vi "Main_FPGA.vi"() -> ()   [LabVIEW 2018]
uses:
  <vilib>/rvi/eio/common/nirviEmuTemplateMethod_errors.vi
  <vilib>/rvi/Emulation/niFpgaGetClockAttributes.vi
  <vilib>/rvi/Emulation/niFpgaSctlEmulationGetInTimedLoop.vi
  <vilib>/rvi/Emulation/niFpgaEmulationReportErrorSimple.vi
  <vilib>/rvi/Emulation/niFpgaProcessEmulError.vi
  <vilib>/rvi/Emulation/niFpgaCriticalErrorInLSC.vi
  <vilib>/eio/EIONode/EIONode.xnode
  <vilib>/addons/control/pid/fpga.llb/XNode/niFpgaPID.xnode
panel:
  in  "Mod7/13 Intercooler in temp":fxp<+/-,20,5>
  out "Mod6/Unit L":bool
  out "Mod6/Unit R":bool
  out "Mod8/AI15":fxp<+/-,24,5>
  out "Mod8/AI5":fxp<+/-,24,5>
  out "Mod8/AI4":fxp<+/-,24,5>
  out "Speed_cmd":fxp<+/-,17,6>
  in  "FeedFw_Ena":bool
  in  "ACC_FeedFw":fxp<+/-,16,5>
  out "Acc_2":fxp<+/-,36,10>
  out "Acc_1":fxp<+/-,36,10>
  in  "E-Acc_2":T1={"Gain"=1.0, "OffSet"=0.0}
  in  "E-Acc_1":T1={"Gain"=1.0, "OffSet"=0.0}
  in  "Speed Control Soll (%)":fxp<+/-,16,5>
  in  "Parameter Speed Control":fxp<+/-,16,5>
  in  "PID gains":T2={"proportional gain (Kc)"=1.5, "integral gain (Kc*Ts/Ti)"=0.19921875, "derivative gain (Kc*Td/Ts)"=0.0}
  in  "output range":T3={"output high"=10.0, "output low"=0.0}
  in  "Regler Speed Control":bool
  in  "Ist Speed Control":fxp<+/-,16,5>
  in  "Count (mSec) Fahrhebel":u32=25
  out "Tick Count(mSec) Hydraulic Wave":u32
  out "Count Hydraulic  Wave":i64
  out "Mod6/Fuel Transmitter":bool
  out "Mod6/DI30":bool
  out "Tick Count(mSec) Hydraulic":u32
  out "Count Hydraulic":i64
  in  "Mod7/Hydraulic clutch Set point":fxp<+/-,20,5>
  in  "Mod7/Hydraulic pump actuator Soll":fxp<+/-,20,5>
  in  "Mod7/Out 2":fxp<+/-,20,5>
  in  "Mod7/Out 1":fxp<+/-,20,5>
  out "DM Count":i64
  out "Tick Count(mSec)":u32
  in  "Mod4/DO30":bool
  in  "Mod4/Release Brake M":bool
  in  "Mod4/Richtung Engine Speed M":bool
  in  "Mod4/Release Engine Speed M":bool
  in  "Mod4/Richtung Up M":bool
  in  "Mod4/Release Up M":bool
  out "Mod6/End Position DOWN M":bool
  out "Mod6/DOWN M":bool
  out "Mod6/UP M":bool
  out "Mod6/End Position UP M":bool
  in  "Mod7/Up M Set point":fxp<+/-,20,5>
  in  "Mod7/Torque M Set point":fxp<+/-,20,5>
  out "Mod8/Engine Speed M":fxp<+/-,24,5>
  out "Mod8/Up M":fxp<+/-,24,5>
  in  "Mod4/Clutch":bool
  in  "Mod4/Temperature Control Release":bool
  in  "Mod4/Temperature Control OFF":bool
  in  "Mod4/Calibration ON Brake H":bool
  in  "Mod4/Unit ON Brake H":bool
  in  "Mod4/Brake Performance ON Brake H":bool
  in  "Mod4/Control Reset Brake H":bool
  in  "Mod4/Control ON Brake H":bool
  in  "Mod4/Oil ON":bool
  in  "Mod3/Calibration Brake R":bool
  in  "Mod3/Unit ON Brake R":bool
  in  "Mod3/Brake Performance ON Brake R":bool
  in  "Mod3/Control Reset Brake R":bool
  in  "Mod3/Control ON Brake R":bool
  in  "Mod3/Horn":bool
  in  "Mod3/DO20":bool
  in  "Mod3/Speed Control Release":bool
  in  "Mod3/DO18":bool
  in  "Mod3/Flashing light":bool
  in  "Mod3/Calibration ON Brake L":bool
  in  "Mod3/Unit ON Brake L":bool
  in  "Mod3/Brake Performance ON Brake L":bool
  in  "Mod3/Control Reset Brake L":bool
  in  "Mod3/Control ON Brake L":bool
  in  "Mod3/Converter Clutch ON":bool
  in  "Mod3/Fuel Pump ON":bool
  in  "Mod3/Engine Ignition ON":bool
  in  "Mod3/Start Engine":bool
  in  "Mod3/Engine Pre Glow ON":bool
  in  "Cooling  Set point (°C)":fxp<+/-,16,5>
  in  "Heater Set point (°C)":fxp<+/-,16,5>
  in  "Alarm 24 ON":bool
  in  "Alarm 23 ON":bool
  in  "Alarm 22 ON":bool
  in  "Alarm 21 ON":bool
  in  "Alarm 20 ON":bool
  in  "Alarm 19 ON":bool
  in  "Alarm 18 ON":bool
  in  "Alarm 17 ON":bool
  in  "Alarm 16 ON":bool
  in  "Alarm 15 ON":bool
  in  "Alarm 14 ON":bool
  in  "Alarm 13 ON":bool
  in  "Alarm 12 ON":bool
  in  "Alarm 11 ON":bool
  in  "Alarm 10 ON":bool
  in  "Alarm 9 ON":bool
  in  "Alarm 8 ON":bool
  in  "Alarm 7 ON":bool
  in  "Alarm 6 ON":bool
  in  "Alarm 5 ON":bool
  in  "Alarm 4 ON":bool
  in  "Alarm 3 ON":bool
  out "Alarm":bool
  in  "Alarm 2 ON":bool
  in  "Alarm 1 ON":bool
  in  "Alarm ON":bool
  in  "STOP":bool
  out "Mod8/Kal 2 Brake H":fxp<+/-,24,5>
  out "Mod8/Kal 1 Brake H":fxp<+/-,24,5>
  out "Mod8/Kal 2 Brake R":fxp<+/-,24,5>
  out "Mod8/Kal 1 Brake R":fxp<+/-,24,5>
  out "Mod8/Kal 2 Brake L":fxp<+/-,24,5>
  out "Mod8/Kal 1 Brake L":fxp<+/-,24,5>
  out "Mod8/Engine Speed Wave Sensor":fxp<+/-,24,5>
  out "Mod8/Speed Control":fxp<+/-,24,5>
  out "Mod8/Torque  H":fxp<+/-,24,5>
  out "Mod8/Torque  R":fxp<+/-,24,5>
  out "Mod8/Torque  L":fxp<+/-,24,5>
  in  "Mod3/System Reset/ON":bool
  out "Mod6/Clutch open":bool
  out "Mod6/Clutch closed":bool
  out "Mod6/Alarm 25 Basement":bool
  out "Mod6/Unit L-R":bool
  out "Mod6/Unit H":bool
  out "Mod6/Unit H-L-R":bool
  out "Mod6/Sytem Ready":bool
  out "Mod6/Watchdog Ready":bool
  out "Mod6/Alarm 2 Brake back":bool
  out "Mod6/Alarm 1 Brake back":bool
  out "Mod6/Temperature Brake back":bool
  out "Mod6/Ready Brake back":bool
  out "Mod6/Error Brake back":bool
  out "Mod6/Alarm 24 Overload Warning Oil Heating":bool
  out "Mod6/Alarm 23 Overload Warning Oil Pump":bool
  out "Mod6/Alarm 22 max Oil Pressure":bool
  out "Mod6/Alarm 21 min Oil Pressure":bool
  out "Mod6/Alarm 20 max Oil Temperature":bool
  out "Mod6/Alarm 18 Oil Level":bool
  out "Mod6/Alarm 19 min Oil Pressure":bool
  out "Mod6/Alarm 17 Oil Pressure Difference":bool
  out "Mod5/Alarm 2 Brake R":bool
  out "Mod5/Alarm 1 Brake R":bool
  out "Mod5/Temperature Brake R":bool
  out "Mod5/Ready Brake R":bool
  out "Mod5/Error Brake R":bool
  out "Mod5/Alarm 16 Fundament 4":bool
  out "Mod5/Alarm 15 Fundament 3":bool
  out "Mod5/Alarm 14 Fundament 2":bool
  out "Mod5/Alarm 13 Fundament 1":bool
  out "Mod5/Alarm 12 Spring Element":bool
  out "Mod5/Alarm 11 Watchdog":bool
  out "Mod5/Alarm 10 Fuel Depot":bool
  out "Mod5/Alarm 9 IGBT_ON":bool
  out "Mod5/Alarm 2 Brake L":bool
  out "Mod5/Alarm 1 Brake L":bool
  out "Mod5/Temperature Brake L":bool
  out "Mod5/Ready Brake L":bool
  out "Mod5/Error Brake L":bool
  out "Mod5/Alarm 8 Cooling Water":bool
  out "Mod5/Alarm 7 Exhaust":bool
  out "Mod5/Alarm 6 CO2":bool
  out "Mod5/Alarm 5 Clutch":bool
  out "Mod5/Alarm 4 Speed Control":bool
  out "Mod5/Alarm 3 Flow Control Unit":bool
  out "Mod5/Alarm 2 Gas":bool
  out "Mod5/Alarm 1 Fire":bool
  out "Mod2/Engine Speed  H":fxp<+/-,20,5>
  out "Mod2/Engine Speed R":fxp<+/-,20,5>
  out "Mod2/Engine Speed  L":fxp<+/-,20,5>
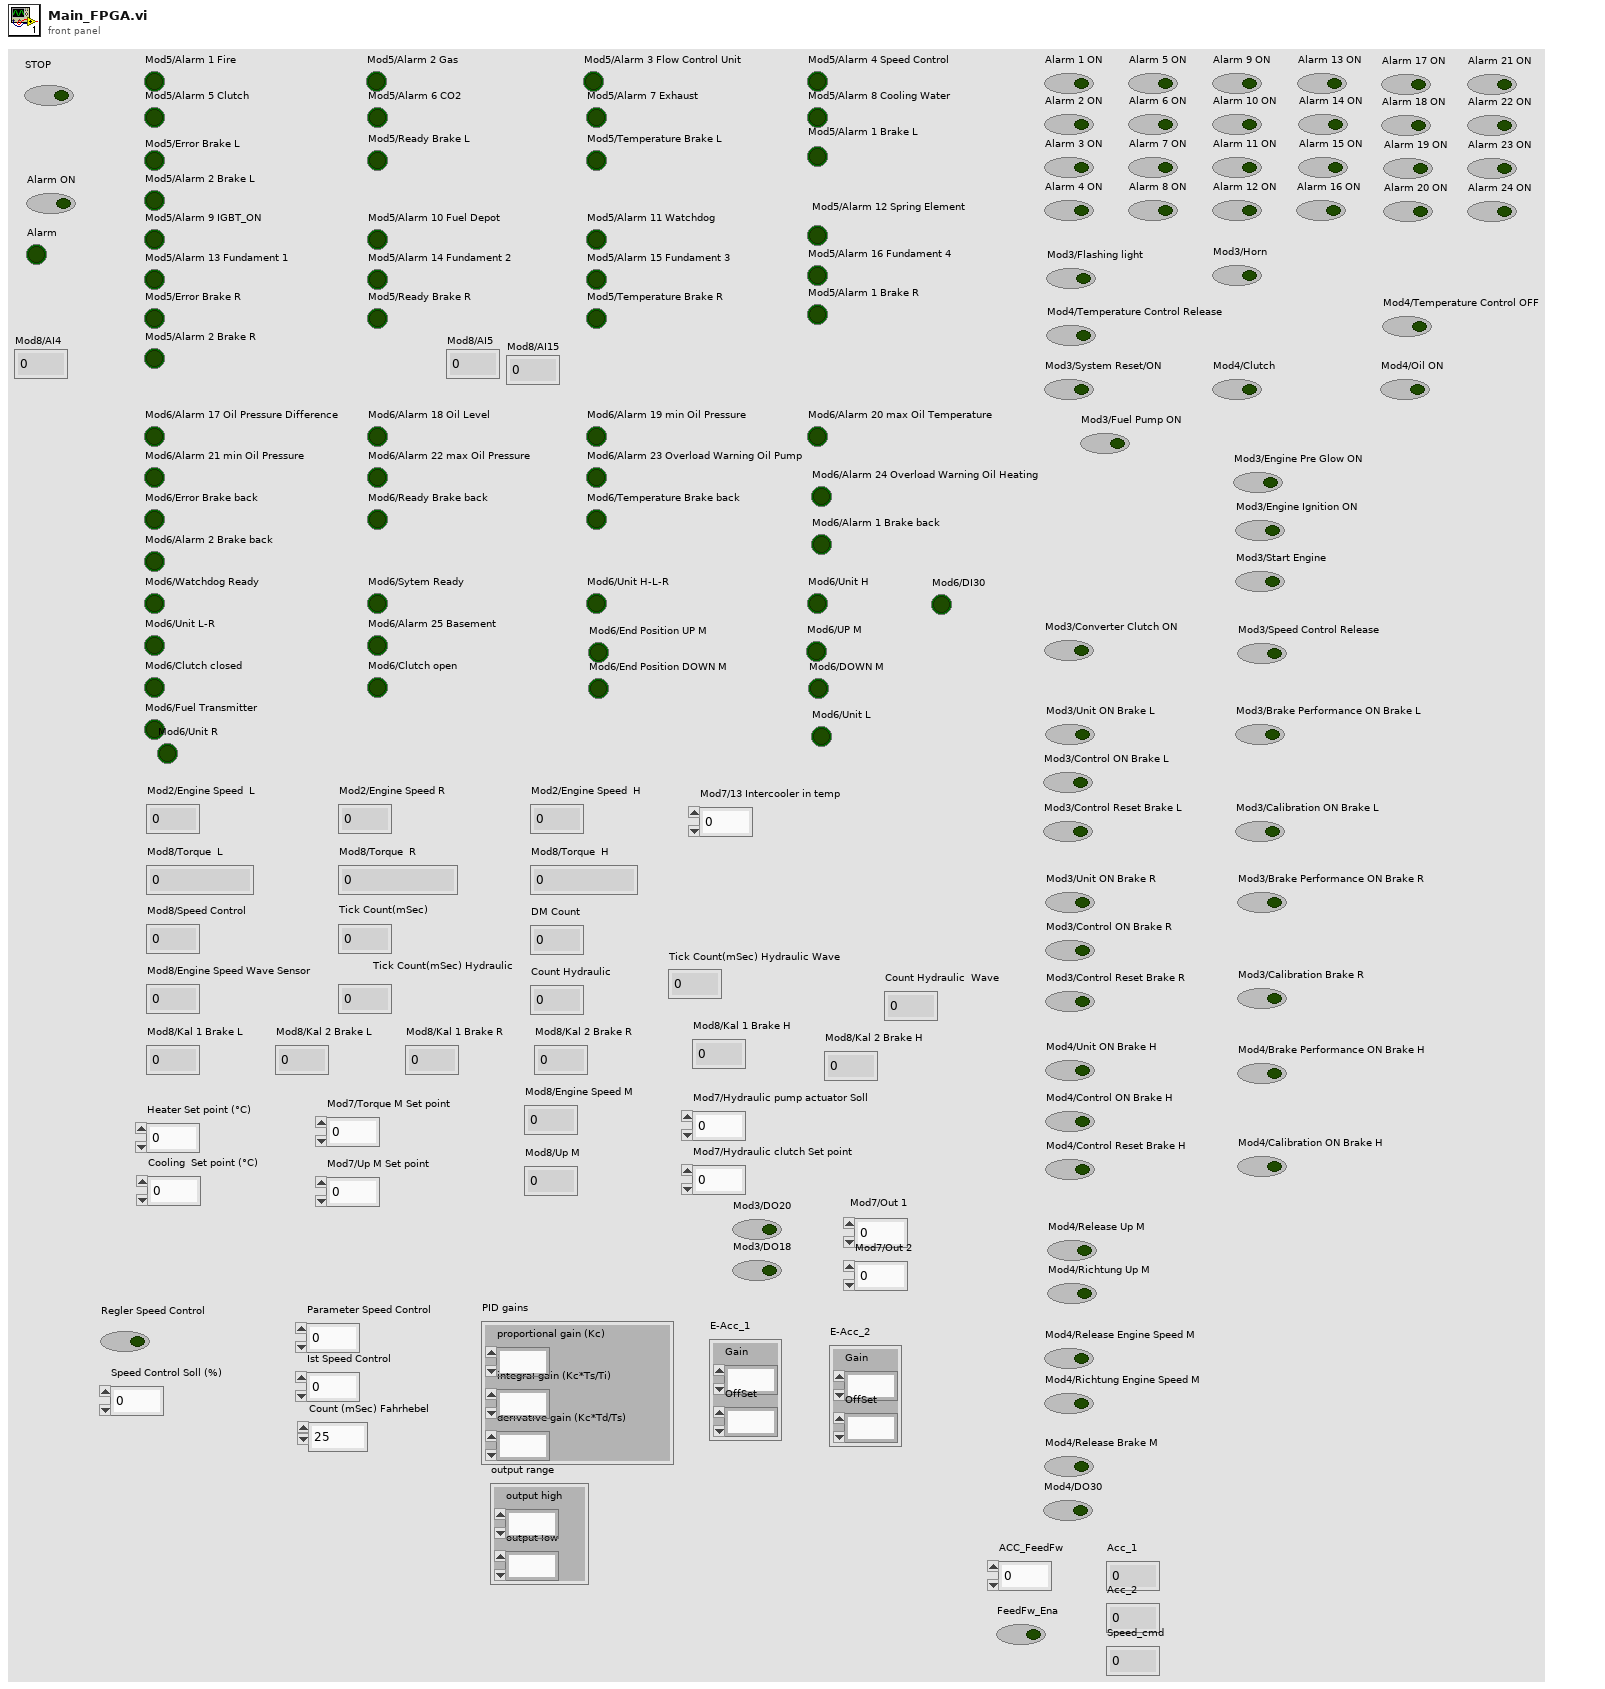
[diagram p1: front panel]
types:
  T1 = cluster{"Gain":fxp<+/-,20,5>, "OffSet":fxp<+/-,20,5>}
  T2 = cluster{"proportional gain (Kc)":fxp<+/-,16,8>, "integral gain (Kc*Ts/Ti)":fxp<+/-,16,8>, "derivative gain (Kc*Td/Ts)":fxp<+/-,16,8>}
  T3 = cluster{"output high":fxp<+/-,16,5>, "output low":fxp<+/-,16,5>}
  T4 = cluster{"proportional gain (Kc)":i16, "integral gain (Kc*Ts/Ti)":i16, "derivative gain (Kc*Td/Ts)":i16}
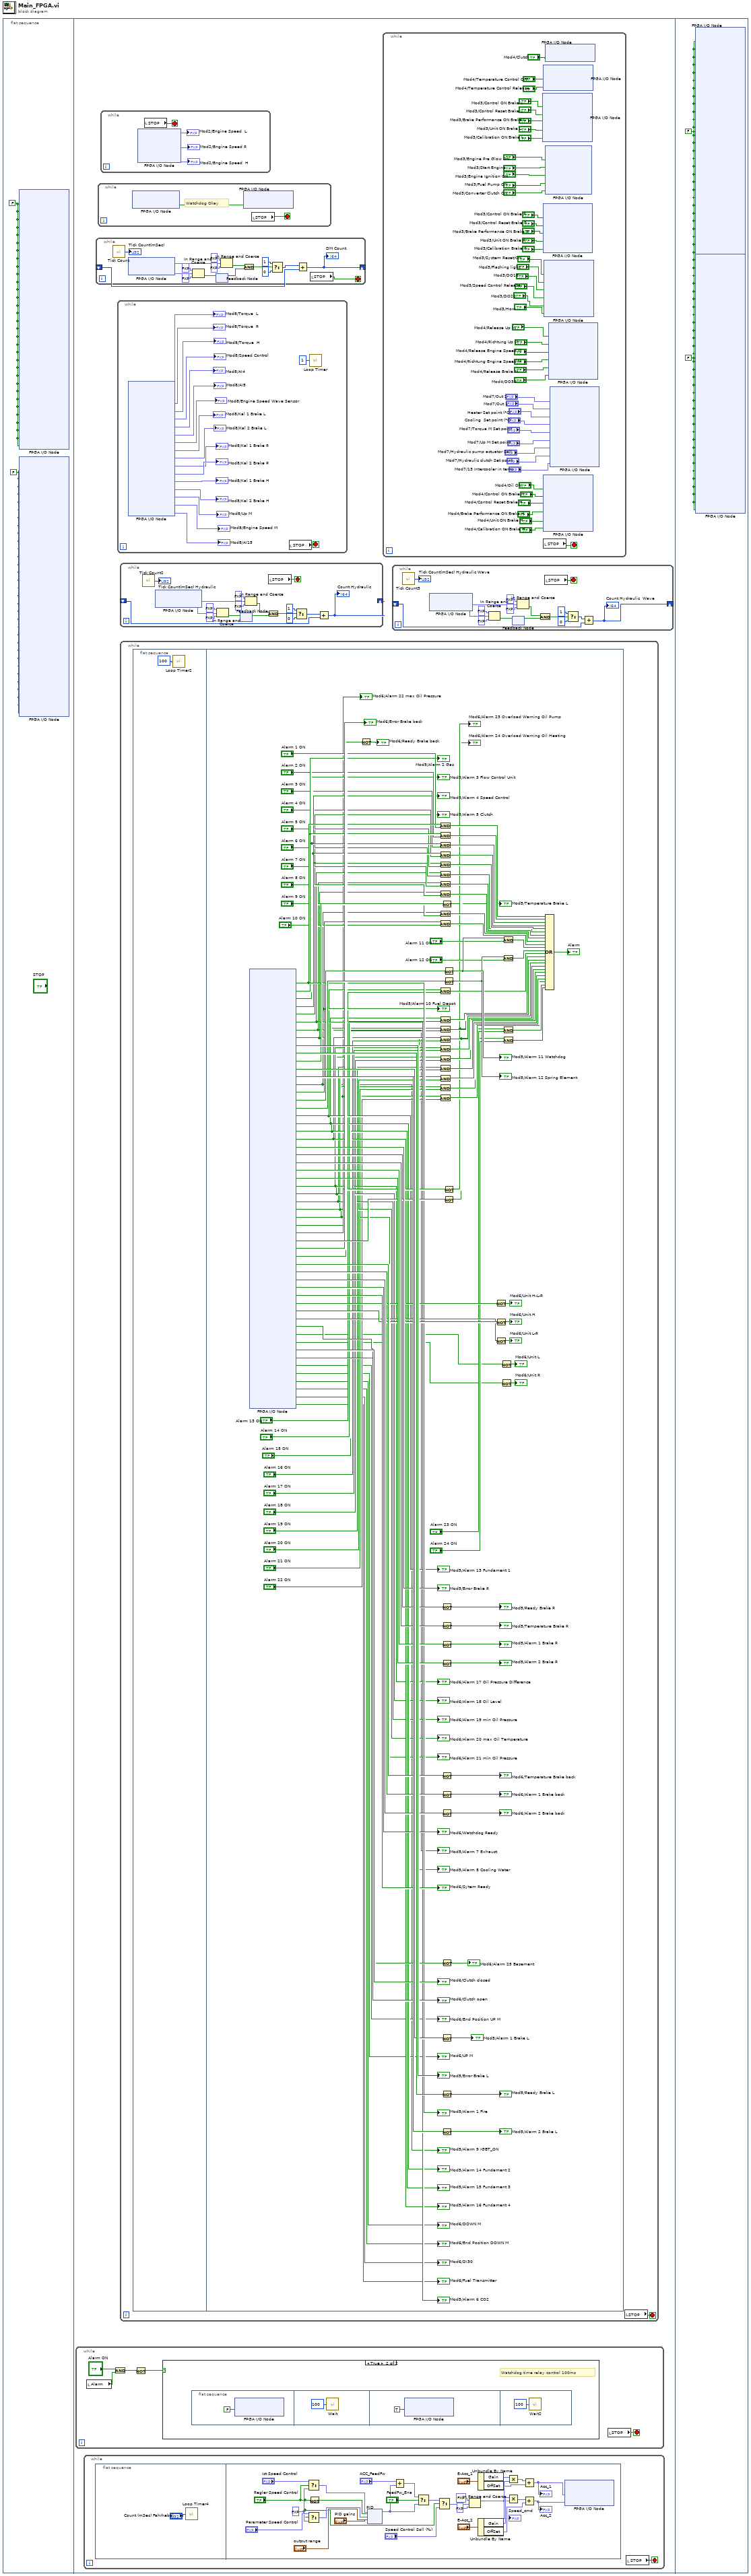
[diagram p0: block diagram]
diagram:
  n1 = flat-sequence {
    frame #0 {
      w1 = FALSE ("Mod4/DO0")
      w2 = FALSE ("Mod3/DO0")
      n2 = xnode "FPGA I/O Node"("Mod4/DO0"=w1, "Mod4/DO1"=w1, "Mod4/DO2"=w1, "Mod4/DO3"=w1, "Mod4/DO4"=w1, "Mod4/DO5"=w1, "Mod4/DO6"=w1, "Mod4/DO7"=w1, "Mod4/DO8"=w1, "Mod4/DO9"=w1, "Mod4/DO10"=w1, "Mod4/DO11"=w1, "Mod4/DO12"=w1, "Mod4/DO13"=w1, "Mod4/DO14"=w1, "Mod4/DO15"=w1, "Mod4/DO16"=w1, "Mod4/DO17"=w1, "Mod4/DO18"=w1, "Mod4/DO19"=w1, "Mod4/DO20"=w1, "Mod4/DO21"=w1, "Mod4/DO22"=w1, "Mod4/DO23"=w1, "Mod4/DO24"=w1, "Mod4/DO25"=w1, "Mod4/DO26"=w1, "Mod4/DO27"=w1, "Mod4/DO28"=w1, "Mod4/DO29"=w1, "Mod4/DO30"=w1, "Mod4/DO31"=w1) -> ()  [unwired: 32 in, 32 out]
      n3 = xnode "FPGA I/O Node"("Mod3/DO0"=w2, "Mod3/DO1"=w2, "Mod3/DO2"=w2, "Mod3/DO3"=w2, "Mod3/DO4"=w2, "Mod3/DO5"=w2, "Mod3/DO6"=w2, "Mod3/DO7"=w2, "Mod3/DO8"=w2, "Mod3/DO9"=w2, "Mod3/DO10"=w2, "Mod3/DO11"=w2, "Mod3/DO12"=w2, "Mod3/DO13"=w2, "Mod3/DO14"=w2, "Mod3/DO15"=w2, "Mod3/DO16"=w2, "Mod3/DO17"=w2, "Mod3/DO18"=w2, "Mod3/DO19"=w2, "Mod3/DO20"=w2, "Mod3/DO21"=w2, "Mod3/DO22"=w2, "Mod3/DO23"=w2, "Mod3/DO24"=w2, "Mod3/DO25"=w2, "Mod3/DO26"=w2, "Mod3/DO27"=w2, "Mod3/DO28"=w2, "Mod3/DO29"=w2, "Mod3/DO30"=w2, "Mod3/DO31"=w2) -> ()  [unwired: 32 in, 32 out]
    }
    frame #1 {
      n4 = while {
        stop <- w178 stop-if-true
        n5 = local read "Alarm"() -> (w181:bool)
        n6 = And(x="Alarm ON", y=w181) -> (x .and. y?=w180:bool)
        n7 = Not(x=w180) -> (.not. x?=w179:bool)
        n8 = case shown="True" w179 {
          frame False {
          }
          frame True {
            # "Watchdog time relay control 100ms"
            n9 = flat-sequence {
              frame #0 {
                n10 = xnode "FPGA I/O Node"("Mod4/DO16"=FALSE) -> ()  [unwired: 1 in, 1 out]
              }
              frame #1 {
                n11 = call "Wait"("Count(mSec)"=u32 100) -> ()  [unwired: 1 out]
              }
              frame #2 {
                n12 = xnode "FPGA I/O Node"("Mod4/DO16"=TRUE) -> ()  [unwired: 1 in, 1 out]
              }
              frame #3 {
                n13 = call "Wait2"("Count(mSec)"=u32 100) -> ()  [unwired: 1 out]
              }
            }
          }
        }
        n14 = local read "STOP"() -> (w178:bool)
      }
      n15 = while {
        stop <- w25 stop-if-true
        n16 = flat-sequence {
          frame #0 {
            n17 = call "Loop Timer4"("Count(mSec)"="Count (mSec) Fahrhebel") -> ()  [unwired: 1 out]
          }
          frame #1 {
            w49 = fxp<+,1,1> 0.0 ("t")
            n18 = Select(t="Ist Speed Control", s="Regler Speed Control", f=w49) -> (s? t:f=w54:fxp<+/-,16,5>)
            n19 = Select(t="Parameter Speed Control", s="Regler Speed Control", f=w49) -> (s? t:f=w53:fxp<+/-,16,5>)
            n20 = Not(x="Regler Speed Control") -> (.not. x?=w48:bool)
            n21 = xnode "PID"("process variable"=w54, "reset?"=w48, "setpoint"=w53, "PID gains"="PID gains", "output range"="output range") -> ("output"=w34:fxp<+/-,16,5>)
            n22 = Add(x="ACC_FeedFw", y=w34) -> (x+y=w35:fxp<+/-,17,6>)
            n23 = Select(t=w35, s="FeedFw_Ena", f=w34) -> (s? t:f=w36:fxp<+/-,17,6>)
            n24 = Select(t=w36, s="Regler Speed Control", f="Speed Control Soll (%)") -> (s? t:f=w30:fxp<+/-,17,6>)
            n25 = In Range and Coerce(upper limit=fxp<+/-,17,6> 10.0, x=w30, lower limit=fxp<+/-,17,6> 0.0) -> (coerced(x)=w29:fxp<+/-,17,6>)  [unwired: 1 out]
            "Speed_cmd" <- w29
            n26 = Unbundle By Name("E-Acc_1") -> ("Gain"=w45:fxp<+/-,20,5>, "OffSet"=w43:fxp<+/-,20,5>)
            n27 = Unbundle By Name("E-Acc_2") -> ("Gain"=w40:fxp<+/-,20,5>, "OffSet"=w39:fxp<+/-,20,5>)
            n28 = Multiply(x=w45, y=w29) -> (x*y=w44:fxp<+/-,37,11>)
            n29 = Multiply(x=w40, y=w29) -> (x*y=w41:fxp<+/-,37,11>)
            n30 = Add(x=w44, y=w43) -> (x+y=w42:fxp<+/-,37,11>)
            "Acc_1" <- w42
            n31 = Add(x=w41, y=w39) -> (x+y=w38:fxp<+/-,37,11>)
            "Acc_2" <- w38
            n32 = xnode "FPGA I/O Node"("Mod7/AO14"=w42, "Mod7/AO15"=w38) -> ()  [unwired: 2 in, 2 out]
          }
        }
        n33 = local read "STOP"() -> (w25:bool)
      }
      n34 = while {
        shift-right: [w124] -> _
        shift-left: _ -> [w125]
        stop <- w122 stop-if-true
        n35 = call "Tick Count"() -> ("Tick Count(mSec)"=→"Tick Count(mSec)":u32)
        n36 = xnode "FPGA I/O Node"() -> ("Mod8/AI14"=w119:fxp<+/-,24,5>)  [unwired: 1 in, 1 out]
        n37 = In Range and Coerce(upper limit=fxp<+/-,24,5> 3.0, x=w119, lower limit=fxp<+/-,24,5> 0.0) -> (In Range?=w120:bool)  [unwired: 1 out]
        n38 = feedback-in #1(w120) -> ()
        n39 = feedback #1() -> (w121:bool)  [unwired: 1 in]
        n40 = In Range and Coerce(upper limit=fxp<+/-,24,5> 6.0, x=w119, lower limit=fxp<+/-,24,5> 3.0) -> (In Range?=w116:bool)  [unwired: 1 out]
        n41 = And(x=w116, y=w121) -> (x .and. y?=w129:bool)
        n42 = Select(t=i64 1, s=w129, f=i64 0) -> (s? t:f=w126:i64)
        n43 = Add(x=w126, y=w125) -> (x+y=w124:i64)
        "DM Count" <- w124
        n44 = local read "STOP"() -> (w122:bool)
      }
      n45 = while {
        stop <- w187 stop-if-true
        # "Watchdog Okay"
        n46 = xnode "FPGA I/O Node"() -> ("Mod6/DI16"=w188:bool)  [unwired: 1 in, 1 out]
        n47 = xnode "FPGA I/O Node"("Mod4/DO17"=w188) -> ()  [unwired: 1 in, 1 out]
        n48 = local read "STOP"() -> (w187:bool)
      }
      n49 = while {
        stop <- w21 stop-if-true
        n50 = xnode "FPGA I/O Node"() -> ("Mod2/AI0"=→"Mod2/Engine Speed  L":fxp<+/-,20,5>, "Mod2/AI1"=→"Mod2/Engine Speed R":fxp<+/-,20,5>, "Mod2/AI2"=→"Mod2/Engine Speed  H":fxp<+/-,20,5>)  [unwired: 3 in, 3 out]
        n51 = local read "STOP"() -> (w21:bool)
      }
      n52 = while {
        stop <- w7 stop-if-true
        n53 = xnode "FPGA I/O Node"() -> ("Mod8/AI0"=→"Mod8/Torque  L":fxp<+/-,24,5>, "Mod8/AI1"=→"Mod8/Torque  R":fxp<+/-,24,5>, "Mod8/AI2"=→"Mod8/Torque  H":fxp<+/-,24,5>, "Mod8/AI3"=→"Mod8/Speed Control":fxp<+/-,24,5>, "Mod8/AI4"=→"Mod8/AI4":fxp<+/-,24,5>, "Mod8/AI5"=→"Mod8/AI5":fxp<+/-,24,5>, "Mod8/AI6"=→"Mod8/Engine Speed Wave Sensor":fxp<+/-,24,5>, "Mod8/AI7"=→"Mod8/Kal 1 Brake L":fxp<+/-,24,5>, "Mod8/AI8"=→"Mod8/Kal 2 Brake L":fxp<+/-,24,5>, "Mod8/AI9"=→"Mod8/Kal 1 Brake R":fxp<+/-,24,5>, "Mod8/AI10"=→"Mod8/Kal 2 Brake R":fxp<+/-,24,5>, "Mod8/AI11"=→"Mod8/Kal 1 Brake H":fxp<+/-,24,5>, "Mod8/AI12"=→"Mod8/Kal 2 Brake H":fxp<+/-,24,5>, "Mod8/AI13"=→"Mod8/Up M":fxp<+/-,24,5>, "Mod8/AI14"=→"Mod8/Engine Speed M":fxp<+/-,24,5>, "Mod8/AI15"=→"Mod8/AI15":fxp<+/-,24,5>)  [unwired: 16 in, 16 out]
        n54 = local read "STOP"() -> (w7:bool)
        n55 = call "Loop Timer"("Count(mSec)"=u32 1) -> ()  [unwired: 1 out]
      }
      n56 = while {
        shift-right: [w108] -> _
        shift-left: _ -> [w109]
        stop <- w106 stop-if-true
        n57 = call "Tick Count2"() -> ("Tick Count(mSec)"=→"Tick Count(mSec) Hydraulic":u32)
        n58 = xnode "FPGA I/O Node"() -> ("Mod8/AI15"=w103:fxp<+/-,24,5>)  [unwired: 1 in, 1 out]
        n59 = In Range and Coerce(upper limit=fxp<+/-,24,5> 3.0, x=w103, lower limit=fxp<+/-,24,5> 0.0) -> (In Range?=w104:bool)  [unwired: 1 out]
        n60 = feedback-in #2(w104) -> ()
        n61 = feedback #2() -> (w105:bool)  [unwired: 1 in]
        n62 = In Range and Coerce(upper limit=fxp<+/-,24,5> 6.0, x=w103, lower limit=fxp<+/-,24,5> 3.0) -> (In Range?=w100:bool)  [unwired: 1 out]
        n63 = And(x=w100, y=w105) -> (x .and. y?=w113:bool)
        n64 = local read "STOP"() -> (w106:bool)
        n65 = Select(t=i64 1, s=w113, f=i64 0) -> (s? t:f=w110:i64)
        n66 = Add(x=w110, y=w109) -> (x+y=w108:i64)
        "Count Hydraulic" <- w108
      }
      n67 = while {
        stop <- w189 stop-if-true
        n68 = flat-sequence {
          frame #0 {
            n69 = call "Loop Timer2"("Count(mSec)"=u32 100) -> ()  [unwired: 1 out]
          }
          frame #1 {
            n70 = xnode "FPGA I/O Node"() -> ("Mod5/DI0"=w277:bool, "Mod5/DI1"=w275:bool, "Mod5/DI2"=w273:bool, "Mod5/DI3"=w266:bool, "Mod5/DI4"=w255:bool, "Mod5/DI5"=w256:bool, "Mod5/DI6"=w196:bool, "Mod5/DI7"=w197:bool, "Mod5/DI8"=→"Mod5/Error Brake L":bool, "Mod5/DI9"=w315:bool, "Mod5/DI10"=w314:bool, "Mod5/DI11"=w313:bool, "Mod5/DI12"=w312:bool, "Mod5/DI16"=w195:bool, "Mod5/DI17"=w252:bool, "Mod5/DI18"=w311:bool, "Mod5/DI19"=w310:bool, "Mod5/DI20"=w243:bool, "Mod5/DI21"=w240:bool, "Mod5/DI22"=w237:bool, "Mod5/DI23"=w234:bool, "Mod5/DI24"=→"Mod5/Error Brake R":bool, "Mod5/DI25"=w304:bool, "Mod5/DI26"=w308:bool, "Mod5/DI27"=w307:bool, "Mod5/DI28"=w306:bool, "Mod6/DI0"=w231:bool, "Mod6/DI1"=w228:bool, "Mod6/DI2"=w225:bool, "Mod6/DI3"=w222:bool, "Mod6/DI4"=w219:bool, "Mod6/DI5"=w216:bool, "Mod6/DI6"=w278:bool, "Mod6/DI7"=w305:bool, "Mod6/DI8"=→"Mod6/Error Brake back":bool, "Mod6/DI9"=w302:bool, "Mod6/DI10"=w301:bool, "Mod6/DI11"=w285:bool, "Mod6/DI12"=w300:bool, "Mod6/DI16"=→"Mod6/Watchdog Ready":bool, "Mod6/DI17"=→"Mod6/Sytem Ready":bool, "Mod6/DI18"=w297:bool, "Mod6/DI19"=w296:bool, "Mod6/DI20"=w295:bool, "Mod6/DI21"=w280:bool, "Mod6/DI22"=w192:bool, "Mod6/DI23"=w191:bool, "Mod6/DI24"=→"Mod6/Clutch closed":bool, "Mod6/DI25"=→"Mod6/Clutch open":bool, "Mod6/DI26"=→"Mod6/End Position UP M":bool, "Mod6/DI27"=→"Mod6/UP M":bool, "Mod6/DI28"=→"Mod6/DOWN M":bool, "Mod6/DI29"=→"Mod6/End Position DOWN M":bool, "Mod6/DI30"=→"Mod6/DI30":bool, "Mod6/DI31"=→"Mod6/Fuel Transmitter":bool)  [unwired: 55 in, 55 out]
            "Mod5/Alarm 1 Fire" <- w277
            "Mod5/Alarm 2 Gas" <- w275
            "Mod5/Alarm 3 Flow Control Unit" <- w273
            "Mod5/Alarm 4 Speed Control" <- w266
            "Mod5/Alarm 5 Clutch" <- w255
            "Mod5/Alarm 6 CO2" <- w256
            "Mod5/Alarm 7 Exhaust" <- w196
            "Mod5/Alarm 8 Cooling Water" <- w197
            "Mod5/Alarm 9 IGBT_ON" <- w195
            "Mod5/Alarm 10 Fuel Depot" <- w252
            "Mod5/Alarm 13 Fundament 1" <- w243
            "Mod5/Alarm 14 Fundament 2" <- w240
            "Mod5/Alarm 15 Fundament 3" <- w237
            "Mod5/Alarm 16 Fundament 4" <- w234
            "Mod6/Alarm 17 Oil Pressure Difference" <- w231
            "Mod6/Alarm 19 min Oil Pressure" <- w225
            "Mod6/Alarm 18 Oil Level" <- w228
            "Mod6/Alarm 20 max Oil Temperature" <- w222
            "Mod6/Alarm 21 min Oil Pressure" <- w219
            "Mod6/Alarm 22 max Oil Pressure" <- w216
            n71 = Not(x=w302) -> (.not. x?=→"Mod6/Ready Brake back":bool)
            n72 = And(x=w277, y="Alarm 1 ON") -> (x .and. y?=w269:bool)
            n73 = And(x=w275, y="Alarm 2 ON") -> (x .and. y?=w270:bool)
            n74 = And(x=w273, y="Alarm 3 ON") -> (x .and. y?=w268:bool)
            n75 = And(x=w266, y="Alarm 4 ON") -> (x .and. y?=w267:bool)
            n76 = And(x=w255, y="Alarm 5 ON") -> (x .and. y?=w263:bool)
            n77 = And(x=w256, y="Alarm 6 ON") -> (x .and. y?=w262:bool)
            n78 = And(x=w196, y="Alarm 7 ON") -> (x .and. y?=w259:bool)
            n79 = And(x=w197, y="Alarm 8 ON") -> (x .and. y?=w257:bool)
            n80 = And(x=w195, y="Alarm 9 ON") -> (x .and. y?=w253:bool)
            n81 = And(x=w252, y="Alarm 10 ON") -> (x .and. y?=w250:bool)
            n82 = And(x=w243, y="Alarm 13 ON") -> (x .and. y?=w241:bool)
            n83 = And(x=w240, y="Alarm 14 ON") -> (x .and. y?=w239:bool)
            n84 = And(x=w237, y="Alarm 15 ON") -> (x .and. y?=w235:bool)
            n85 = And(x=w234, y="Alarm 16 ON") -> (x .and. y?=w233:bool)
            n86 = And(x=w231, y="Alarm 17 ON") -> (x .and. y?=w229:bool)
            n87 = And(x=w228, y="Alarm 18 ON") -> (x .and. y?=w226:bool)
            n88 = And(x=w225, y="Alarm 19 ON") -> (x .and. y?=w223:bool)
            n89 = And(x=w222, y="Alarm 20 ON") -> (x .and. y?=w220:bool)
            n90 = And(x=w219, y="Alarm 21 ON") -> (x .and. y?=w217:bool)
            n91 = And(x=w216, y="Alarm 22 ON") -> (x .and. y?=w214:bool)
            n92 = Not(x=w314) -> (.not. x?=→"Mod5/Temperature Brake L":bool)
            n93 = Not(x=w304) -> (.not. x?=→"Mod5/Ready Brake R":bool)
            n94 = Not(x=w308) -> (.not. x?=→"Mod5/Temperature Brake R":bool)
            n95 = Not(x=w307) -> (.not. x?=→"Mod5/Alarm 1 Brake R":bool)
            n96 = Not(x=w306) -> (.not. x?=→"Mod5/Alarm 2 Brake R":bool)
            n97 = Not(x=w301) -> (.not. x?=→"Mod6/Temperature Brake back":bool)
            n98 = Not(x=w285) -> (.not. x?=→"Mod6/Alarm 1 Brake back":bool)
            n99 = Not(x=w300) -> (.not. x?=→"Mod6/Alarm 2 Brake back":bool)
            n100 = Not(x=w280) -> (.not. x?=→"Mod6/Alarm 25 Basement":bool)
            n101 = Not(x=w313) -> (.not. x?=→"Mod5/Alarm 1 Brake L":bool)
            n102 = Not(x=w315) -> (.not. x?=→"Mod5/Ready Brake L":bool)
            n103 = Not(x=w312) -> (.not. x?=→"Mod5/Alarm 2 Brake L":bool)
            n104 = Not(x=w311) -> (.not. x?=w249:bool)
            "Mod5/Alarm 11 Watchdog" <- w249
            n105 = Not(x=w310) -> (.not. x?=w246:bool)
            "Mod5/Alarm 12 Spring Element" <- w246
            n106 = Not(x=w278) -> (.not. x?=w213:bool)
            "Mod6/Alarm 23 Overload Warning Oil Pump" <- w213
            n107 = Not(x=w305) -> (.not. x?=w210:bool)
            "Mod6/Alarm 24 Overload Warning Oil Heating" <- w210
            n108 = Not(x=w297) -> (.not. x?=→"Mod6/Unit H-L-R":bool)
            n109 = Not(x=w296) -> (.not. x?=→"Mod6/Unit H":bool)
            n110 = Not(x=w295) -> (.not. x?=→"Mod6/Unit L-R":bool)
            n111 = Not(x=w192) -> (.not. x?=→"Mod6/Unit L":bool)
            n112 = Not(x=w191) -> (.not. x?=→"Mod6/Unit R":bool)
            n113 = And(x=w249, y="Alarm 11 ON") -> (x .and. y?=w247:bool)
            n114 = And(x=w246, y="Alarm 12 ON") -> (x .and. y?=w244:bool)
            n115 = And(x=w213, y="Alarm 23 ON") -> (x .and. y?=w211:bool)
            n116 = And(x=w210, y="Alarm 24 ON") -> (x .and. y?=w208:bool)
            n117 = Compound Arithmetic op=OR(w269, w270, w268, w267, w263, w262, w259, w257, w253, w250, w247, w244, w241, w239, w235, w233, w229, w226, w223, w220, w217, w214, w211, w208) -> (→"Alarm":bool)
          }
        }
        n118 = local read "STOP"() -> (w189:bool)
      }
      n119 = while {
        stop <- w177 stop-if-true
        n120 = xnode "FPGA I/O Node"("Mod3/DO8"="Mod3/Control ON Brake L", "Mod3/DO9"="Mod3/Control Reset Brake L", "Mod3/DO10"="Mod3/Brake Performance ON Brake L", "Mod3/DO11"="Mod3/Unit ON Brake L", "Mod3/DO12"="Mod3/Calibration ON Brake L") -> ()  [unwired: 5 in, 5 out]
        n121 = xnode "FPGA I/O Node"("Mod3/DO24"="Mod3/Control ON Brake R", "Mod3/DO25"="Mod3/Control Reset Brake R", "Mod3/DO26"="Mod3/Brake Performance ON Brake R", "Mod3/DO27"="Mod3/Unit ON Brake R", "Mod3/DO28"="Mod3/Calibration Brake R") -> ()  [unwired: 5 in, 5 out]
        n122 = xnode "FPGA I/O Node"("Mod4/DO18"="Mod4/Temperature Control OFF", "Mod4/DO19"="Mod4/Temperature Control Release") -> ()  [unwired: 2 in, 2 out]
        n123 = xnode "FPGA I/O Node"("Mod4/DO5"="Mod4/Oil ON", "Mod4/DO8"="Mod4/Control ON Brake H", "Mod4/DO9"="Mod4/Control Reset Brake H", "Mod4/DO10"="Mod4/Brake Performance ON Brake H", "Mod4/DO11"="Mod4/Unit ON Brake H", "Mod4/DO12"="Mod4/Calibration ON Brake H") -> ()  [unwired: 6 in, 6 out]
        n124 = local read "STOP"() -> (w177:bool)
        n125 = xnode "FPGA I/O Node"("Mod3/DO16"="Mod3/System Reset/ON", "Mod3/DO17"="Mod3/Flashing light", "Mod3/DO18"="Mod3/DO18", "Mod3/DO19"="Mod3/Speed Control Release", "Mod3/DO20"="Mod3/DO20", "Mod3/DO21"="Mod3/Horn") -> ()  [unwired: 6 in, 6 out]
        n126 = xnode "FPGA I/O Node"("Mod4/DO24"="Mod4/Clutch") -> ()  [unwired: 1 in, 1 out]
        n127 = xnode "FPGA I/O Node"("Mod3/DO0"="Mod3/Engine Pre Glow ON", "Mod3/DO1"="Mod3/Start Engine", "Mod3/DO2"="Mod3/Engine Ignition ON", "Mod3/DO3"="Mod3/Fuel Pump ON", "Mod3/DO4"="Mod3/Converter Clutch ON") -> ()  [unwired: 5 in, 5 out]
        n128 = xnode "FPGA I/O Node"("Mod4/DO25"="Mod4/Release Up M", "Mod4/DO26"="Mod4/Richtung Up M", "Mod4/DO27"="Mod4/Release Engine Speed M", "Mod4/DO28"="Mod4/Richtung Engine Speed M", "Mod4/DO29"="Mod4/Release Brake M", "Mod4/DO30"="Mod4/DO30") -> ()  [unwired: 6 in, 6 out]
        n129 = xnode "FPGA I/O Node"("Mod7/AO2"="Mod7/Out 2", "Mod7/AO1"="Mod7/Out 1", "Mod7/AO3"="Heater Set point (°C)", "Mod7/AO4"="Cooling  Set point (°C)", "Mod7/AO5"="Mod7/Torque M Set point", "Mod7/AO6"="Mod7/Up M Set point", "Mod7/AO7"="Mod7/Hydraulic pump actuator Soll", "Mod7/AO8"="Mod7/Hydraulic clutch Set point", "Mod7/AO13"="Mod7/13 Intercooler in temp") -> ()  [unwired: 9 in, 9 out]
      }
      n130 = while {
        shift-right: [w92] -> _
        shift-left: _ -> [w93]
        stop <- w90 stop-if-true
        n131 = call "Tick Count3"() -> ("Tick Count(mSec)"=→"Tick Count(mSec) Hydraulic Wave":u32)
        n132 = xnode "FPGA I/O Node"() -> ("Mod2/AI3"=w87:fxp<+/-,20,5>)  [unwired: 1 in, 1 out]
        n133 = In Range and Coerce(upper limit=fxp<+/-,24,5> 3.0, x=w87, lower limit=fxp<+/-,24,5> 0.0) -> (In Range?=w88:bool)  [unwired: 1 out]
        n134 = feedback-in #3(w88) -> ()
        n135 = feedback #3() -> (w89:bool)  [unwired: 1 in]
        n136 = In Range and Coerce(upper limit=fxp<+/-,20,5> 6.0, x=w87, lower limit=fxp<+/-,20,5> 3.0) -> (In Range?=w84:bool)  [unwired: 1 out]
        n137 = And(x=w84, y=w89) -> (x .and. y?=w97:bool)
        n138 = local read "STOP"() -> (w90:bool)
        n139 = Select(t=i64 1, s=w97, f=i64 0) -> (s? t:f=w94:i64)
        n140 = Add(x=w94, y=w93) -> (x+y=w92:i64)
        "Count Hydraulic  Wave" <- w92
      }
    }
    frame #2 {
      w317 = FALSE ("Mod4/DO0")
      w318 = FALSE ("Mod3/DO0")
      n141 = xnode "FPGA I/O Node"("Mod4/DO0"=w317, "Mod4/DO1"=w317, "Mod4/DO2"=w317, "Mod4/DO3"=w317, "Mod4/DO4"=w317, "Mod4/DO5"=w317, "Mod4/DO6"=w317, "Mod4/DO7"=w317, "Mod4/DO8"=w317, "Mod4/DO9"=w317, "Mod4/DO10"=w317, "Mod4/DO11"=w317, "Mod4/DO12"=w317, "Mod4/DO13"=w317, "Mod4/DO14"=w317, "Mod4/DO15"=w317, "Mod4/DO16"=w317, "Mod4/DO17"=w317, "Mod4/DO18"=w317, "Mod4/DO19"=w317, "Mod4/DO20"=w317, "Mod4/DO21"=w317, "Mod4/DO22"=w317, "Mod4/DO23"=w317, "Mod4/DO24"=w317, "Mod4/DO25"=w317, "Mod4/DO26"=w317, "Mod4/DO27"=w317, "Mod4/DO28"=w317, "Mod4/DO29"=w317, "Mod4/DO30"=w317, "Mod4/DO31"=w317) -> ()  [unwired: 32 in, 32 out]
      n142 = xnode "FPGA I/O Node"("Mod3/DO0"=w318, "Mod3/DO1"=w318, "Mod3/DO2"=w318, "Mod3/DO3"=w318, "Mod3/DO4"=w318, "Mod3/DO5"=w318, "Mod3/DO6"=w318, "Mod3/DO7"=w318, "Mod3/DO8"=w318, "Mod3/DO9"=w318, "Mod3/DO10"=w318, "Mod3/DO11"=w318, "Mod3/DO12"=w318, "Mod3/DO13"=w318, "Mod3/DO14"=w318, "Mod3/DO15"=w318, "Mod3/DO16"=w318, "Mod3/DO17"=w318, "Mod3/DO18"=w318, "Mod3/DO19"=w318, "Mod3/DO20"=w318, "Mod3/DO21"=w318, "Mod3/DO22"=w318, "Mod3/DO23"=w318, "Mod3/DO24"=w318, "Mod3/DO25"=w318, "Mod3/DO26"=w318, "Mod3/DO27"=w318, "Mod3/DO28"=w318, "Mod3/DO29"=w318, "Mod3/DO30"=w318, "Mod3/DO31"=w318) -> ()  [unwired: 32 in, 32 out]
    }
  }
